vi "Funkcja korelacji.vi"(9 "Sygnal 2":dbl[](array[numeric]), 10 "Sygnal 1":dbl[](array[numeric]), 11 "m":dbl) -> (3 "Funkcja korelacji":dbl)   [LabVIEW 2019]
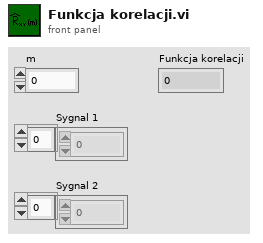
[diagram p1: front panel]
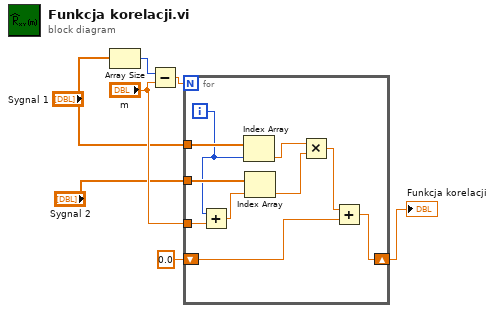
[diagram p0: block diagram]
diagram:
  n1 = Array Size(array="Sygnal 1") -> (size(s)=w3:i32)
  n2 = Subtract(x=w3, y="m") -> (x-y=w2:dbl)
  n3 = for {
    N: w2 -> [_]
    tunnel: "Sygnal 1" -> [w17]
    tunnel: "Sygnal 2" -> [w16]
    tunnel: "m" -> [w13]
    shift-right: [w10] -> w7
    shift-left: 0.0 -> [w8]
    i -> [w14]
    n4 = Add(x=w14, y=w13) -> (x+y=w15:dbl)
    n5 = Index Array(array=w17, index=w14) -> (element=w12:dbl)
    n6 = Index Array(array=w16, index=w15) -> (element=w11:dbl)
    n7 = Multiply(x=w12, y=w11) -> (x*y=w9:dbl)
    n8 = Add(x=w9, y=w8) -> (x+y=w10:dbl)
  }
  "Funkcja korelacji" <- w7
